vi "PCI-USB_DAQ Data Type Cluster .vi"() -> (8 "DO":T1)   [LabVIEW 2015]
uses:
  Digital out.ctl
  Digital out put.ctl
panel:
  in  "DO":T2
  out "Array":string[](array[string])
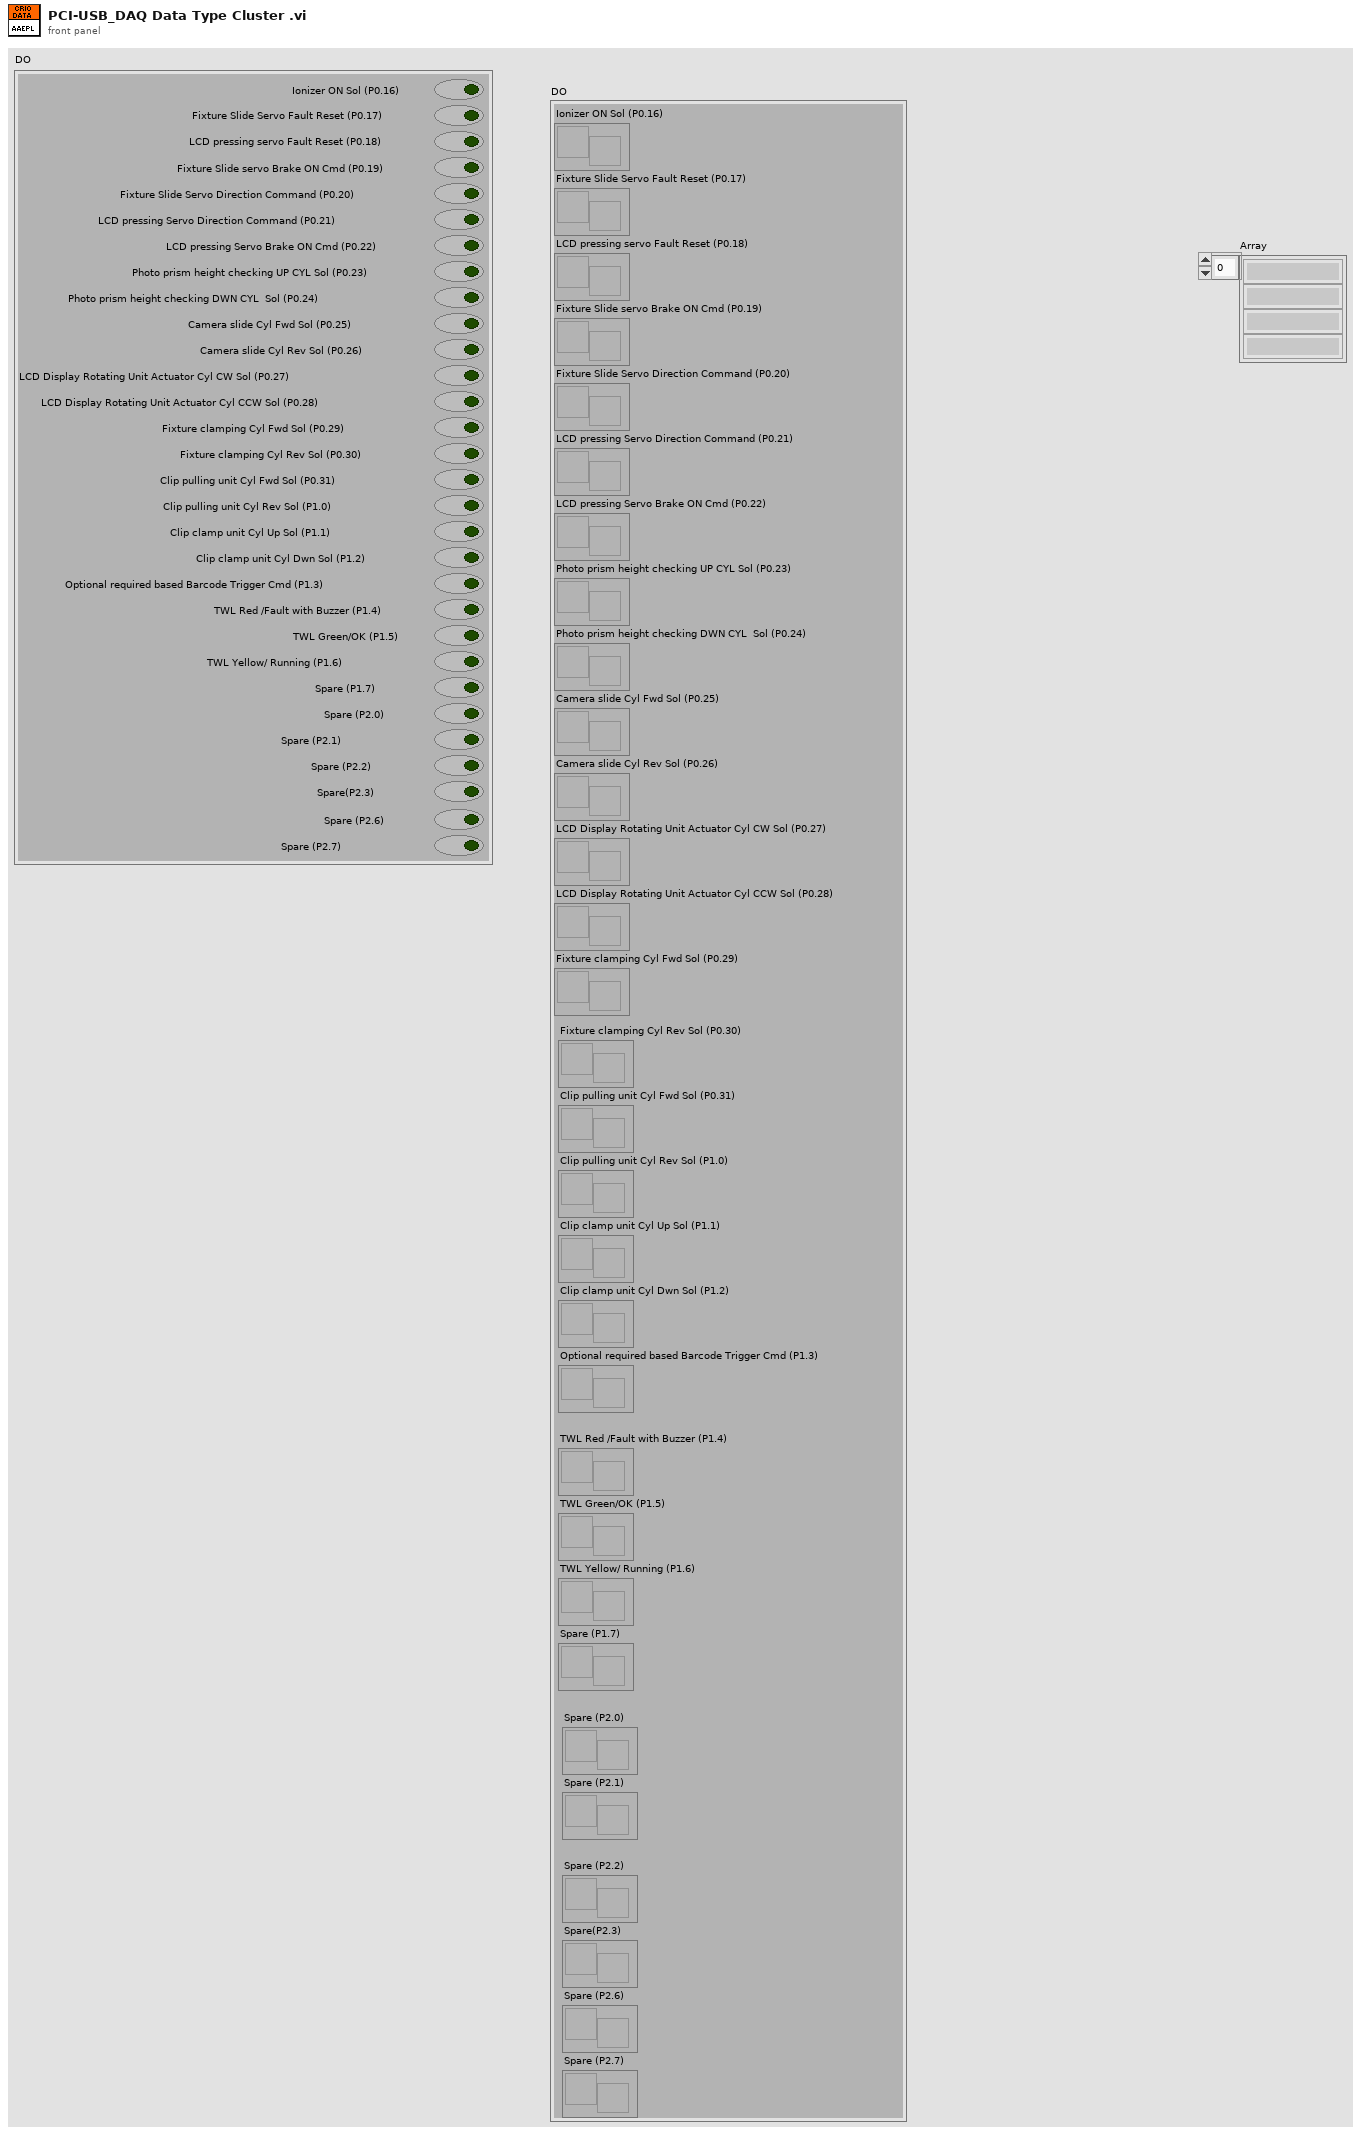
[diagram p1: front panel]
types:
  T1 = typedef "Digital out put.ctl" = cluster{"Ionizer ON Sol (P0.16)":refnum<notifier>, "Fixture Slide Servo Fault Reset (P0.17)":refnum<notifier>, "LCD pressing servo Fault Reset (P0.18)":refnum<notifier>, "Fixture Slide servo Brake ON Cmd (P0.19)":refnum<notifier>, "Fixture Slide Servo Direction Command (P0.20)":refnum<notifier>, "LCD pressing Servo Direction Command (P0.21)":refnum<notifier>, "LCD pressing Servo Brake ON Cmd (P0.22)":refnum<notifier>, "Photo prism height checking UP CYL Sol (P0.23)":refnum<notifier>, "Photo prism height checking DWN CYL  Sol (P0.24)":refnum<notifier>, "Camera slide Cyl Fwd Sol (P0.25)":refnum<notifier>, "Camera slide Cyl Rev Sol (P0.26)":refnum<notifier>, "LCD Display Rotating Unit Actuator Cyl CW Sol (P0.27)":refnum<notifier>, "LCD Display Rotating Unit Actuator Cyl CCW Sol (P0.28)":refnum<notifier>, "Fixture clamping Cyl Fwd Sol (P0.29)":refnum<notifier>, "Fixture clamping Cyl Rev Sol (P0.30)":refnum<notifier>, "Clip pulling unit Cyl Fwd Sol (P0.31)":refnum<notifier>, "Clip pulling unit Cyl Rev Sol (P1.0)":refnum<notifier>, "Clip clamp unit Cyl Up Sol (P1.1)":refnum<notifier>, "Clip clamp unit Cyl Dwn Sol (P1.2)":refnum<notifier>, "Optional required based Barcode Trigger Cmd (P1.3)":refnum<notifier>, "TWL Red /Fault with Buzzer (P1.4)":refnum<notifier>, "TWL Green/OK (P1.5)":refnum<notifier>, "TWL Yellow/ Running (P1.6)":refnum<notifier>, "Spare (P1.7)":refnum<notifier>, "Spare (P2.0)":refnum<notifier>, "Spare (P2.1)":refnum<notifier>, "Spare (P2.2)":refnum<notifier>, "Spare(P2.3)":refnum<notifier>, "Spare (P2.6)":refnum<notifier>, "Spare (P2.7) ":refnum<notifier>}
  T2 = typedef "Digital out.ctl" = cluster{"P2.3-Ok Green":bool, "P1.0-Front cyl fwd sol":bool, "P1.1-Slide cyl fwd ":bool, "P1.2-Slide cyl rev":bool, "P1.3-Left winker":bool, "P1.4-Rh Winker cyl fwd":bool, "P1.5-Cancel cyl fwd":bool, "P1.6-Dipper Rotary cyl fwd":bool, "P1.7-Dipper Rotary cyl Rev":bool, "P2.0-Horn cyl fwd":bool, "P2.1-Passing Cyl fwd":bool, "P2.2-Stamping Cyl  Up":bool, "P2.4-NG Red/buzzer":bool, "P2.5-Heater On cmd":bool, "P1.0-Front cyl fwd sol 2":bool, "P1.1-Slide cyl fwd  2":bool, "P1.2-Slide cyl rev 2":bool, "P1.3-Left winker 2":bool, "P1.4-Rh Winker cyl fwd 2":bool, "P1.5-Cancel cyl fwd 2":bool, "P1.6-Dipper Rotary cyl fwd 2":bool, "P1.7-Dipper Rotary cyl Rev 2":bool, "P2.0-Horn cyl fwd 2":bool, "P2.1-Passing Cyl fwd 2":bool, "P2.2-Stamping Cyl  Up 2":bool, "P2.3-Ok Green 2":bool, "P2.4-NG Red/buzzer 2":bool, "P2.5-Heater On cmd 2":bool, "P2.2-Stamping Cyl  Up 3":bool, "P2.3-Ok Green 3":bool}
  T3 = cluster{"[0]":refnum<notifier>, "[1]":refnum<notifier>, "[2]":refnum<notifier>, "[3]":refnum<notifier>, "[4]":refnum<notifier>, "[5]":refnum<notifier>, "[6]":refnum<notifier>, "[7]":refnum<notifier>, "[8]":refnum<notifier>, "[9]":refnum<notifier>, "[10]":refnum<notifier>, "[11]":refnum<notifier>, "[12]":refnum<notifier>, "[13]":refnum<notifier>, "[14]":refnum<notifier>, "[15]":refnum<notifier>, "[16]":refnum<notifier>, "[17]":refnum<notifier>, "[18]":refnum<notifier>, "[19]":refnum<notifier>, "[20]":refnum<notifier>, "[21]":refnum<notifier>, "[22]":refnum<notifier>, "[23]":refnum<notifier>, "[24]":refnum<notifier>, "[25]":refnum<notifier>, "[26]":refnum<notifier>, "[27]":refnum<notifier>, "[28]":refnum<notifier>, "[29]":refnum<notifier>}
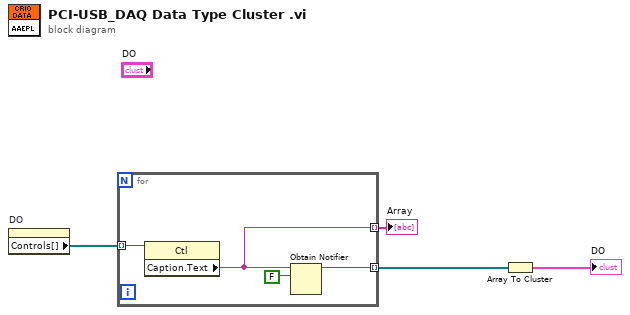
[diagram p0: block diagram]
diagram:
  n1 = property on="DO" class="Clust (strict)"() -> ("Controls[]"=w2:refnum<vi>[])  [unwired: 2 in, 2 out]
  n2 = for {
    tunnel: w2 -> [w8] mode=indexing
    tunnel: [w6] -> w4 mode=indexing
    tunnel: [w5] -> w3 mode=indexing
    n3 = property class="Ctl"(reference=w8) -> ("Caption.Text"=w5:string)  [unwired: 1 in, 2 out]
    n4 = Obtain Notifier(name (unnamed)=w5, notification data type=FALSE) -> (notifier out=w6:refnum<notifier>)  [unwired: 2 in, 2 out]
  }
  "Array" <- w3
  n5 = Array To Cluster(array=w4) -> (cluster=→"DO":T3)
